vi "String - Decode Status.vi"(10 "Status Response String":string) -> (0 "error out":errorcluster, 2 "Module Carrier Status":T1)   [LabVIEW 2017, in "Communications Library.lvlib"]
doc: "Decodes the status response string;\n\nField 0 - State;\n0 - Idle\n1 - Arm\n2 - Run_Pre\n3 - Run_Post\n4 - Post_Process\n5 - Cleanup\n\nField 1 - PreCount - Samples in pre buffer\nField 2 - PostCount - Sample in post buffer\nField 3 - TotalCount - Total samples\nField 4 - Demux Status - Post process status indicator"
uses:
  Communications Library.lvlib
  Typedefs/DTACQ Module Carrier Status.ctl
  Typedefs/DTACQ Status--Enum.ctl
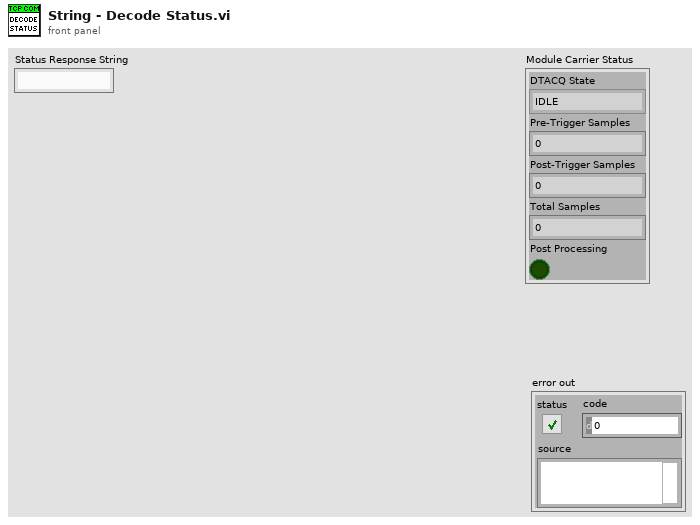
[diagram p1: front panel]
types:
  T1 = typedef "Communications Library.lvlib/DTACQ Module Carrier Status.ctl" = cluster{"DTACQ State":T2, "Pre-Trigger Samples":i32, "Post-Trigger Samples":i32, "Total Samples":i32, "Post Processing":bool}
  T2 = typedef "Communications Library.lvlib/DTACQ Status--Enum.ctl" = enum16{"IDLE", "ARM", "RUN_PRE-TRIGGER", "RUN_POST-TRIGGER", "POST_PROCESS", "CLEANUP"}
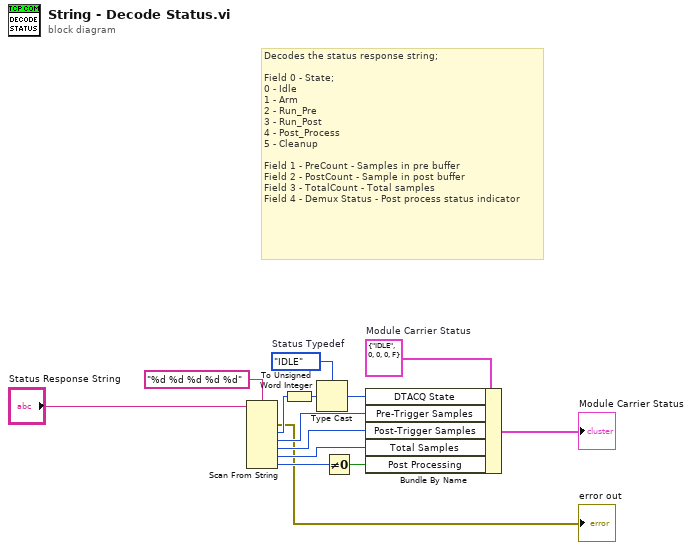
[diagram p0: block diagram]
diagram:
  w6 = T1 {"DTACQ State"=enum."IDLE", "Pre-Trigger Samples"=0, "Post-Trigger Samples"=0, "Total Samples"=0, "Post Processing"=FALSE}  # Module Carrier Status
  w4 = DTACQ_Status--Enum."IDLE"  # Status Typedef
  # "Decodes the status response string;\n\nField 0 - State;\n0 - Idle\n1 - Arm\n2 - Run_Pre\n3 - Run_Post\n4 - Post_Process\n5 - Cleanup\n\nField 1 - PreCount - Samples in pre buffer\nField 2 - PostCount - Sample in post buffer\nField 3 - TotalCount - Total samples\nField 4 - Demux Status - Post process status indicator"
  n1 = Scan From String(format string="%d %d %d %d %d", input string="Status Response String") -> (error out=→"error out":errorcluster, output 1=w13:i32, output 2=w8:i32, output 3=w9:i32, output 4=w10:i32, output 5=w5:i32)  [unwired: 7 in, 2 out]
  n2 = To Unsigned Word Integer(number=w13) -> (unsigned 16bit integer=w14:u16)
  n3 = Type Cast(type=w4, x=w14) -> (*(type *) &x=w7:T2)
  n4 = Not Equal To 0?(x=w5) -> (x != 0?=w11:bool)
  n5 = Bundle By Name(cluster=w6, "DTACQ State"=w7, "Pre-Trigger Samples"=w8, "Post-Trigger Samples"=w9, "Total Samples"=w10, "Post Processing"=w11) -> (→"Module Carrier Status":T1)
